vi "Get Site Info.vi"(8 "Error In":errorcluster, 11 "WebView in":refnum<class "WebView.lvclass">) -> (0 "Error Out":errorcluster, 2 "Site Info":T1, 3 "WebView out":refnum<class "WebView.lvclass">)   [LabVIEW 2024, in "WebView.lvclass"]
uses:
  WebView.lvclass
  WebView.lvclass/WebView.ctl
  <vilib>/sklein/WebView2/Libs/Microsoft.Web.WebView2.Core.dll
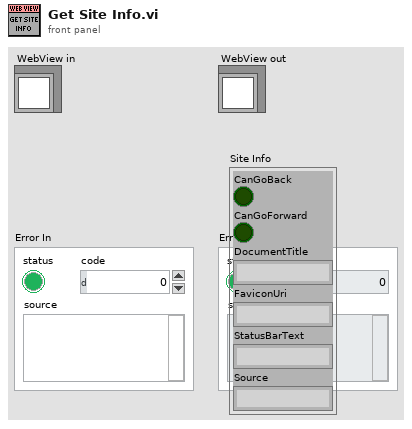
[diagram p1: front panel]
types:
  T1 = cluster{"CanGoBack":bool, "CanGoForward":bool, "DocumentTitle":string, "FaviconUri":string, "StatusBarText":string, "Source":string}
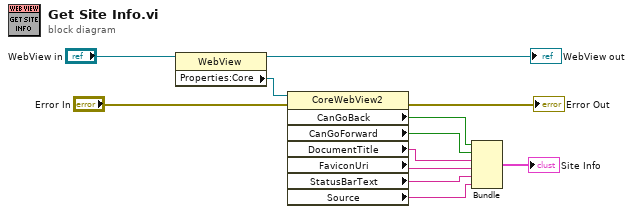
[diagram p0: block diagram]
diagram:
  n1 = property class="WebView"(reference="WebView in") -> (reference out=→"WebView out":refnum<class "WebView.lvclass">, "Properties:Core"=w5:refnum<k24>)  [unwired: 1 in, 1 out]
  n2 = property class="CoreWebView2"(reference=w5, error in="Error In") -> (error out=→"Error Out":errorcluster, "CanGoBack"=w10:bool, "CanGoForward"=w9:bool, "DocumentTitle"=w8:string, "FaviconUri"=w7:string, "StatusBarText"=w4:string, "Source"=w3:string)  [unwired: 1 out]
  n3 = Bundle("CanGoBack"=w10, "CanGoForward"=w9, "DocumentTitle"=w8, "FaviconUri"=w7, "StatusBarText"=w4, "Source"=w3) -> (→"Site Info":T1)  [unwired: 1 in]
